vi "Initialize.vi"(8 "error in (no error)":errorcluster, 9 "GRR Data Mgr":string, 10 "Test Data Mgr":string, 11 "Result Display in":refnum<class "Result Display.lvclass">) -> (0 "error out":errorcluster, 3 "Result Display out":refnum<class "Result Display.lvclass">)   [LabVIEW 2018, in "Result Display.lvclass"]
uses:
  Result Display.lvclass
  Result Display.lvclass/Result Display.ctl
  TestDataMgr/TestDataMgr.lvclass
  Result Data Mgr/Result Data Mgr.lvclass
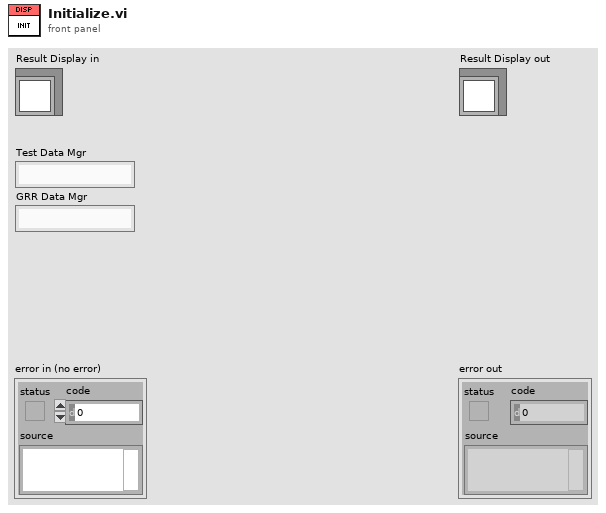
[diagram p1: front panel]
types:
  T1 = typedef "TestDataMgr.lvclass/Session Handle.ctl" = refnum<data-value>
  T2 = typedef "Result Data Mgr.lvclass/Session Handle.ctl" = refnum<data-value>
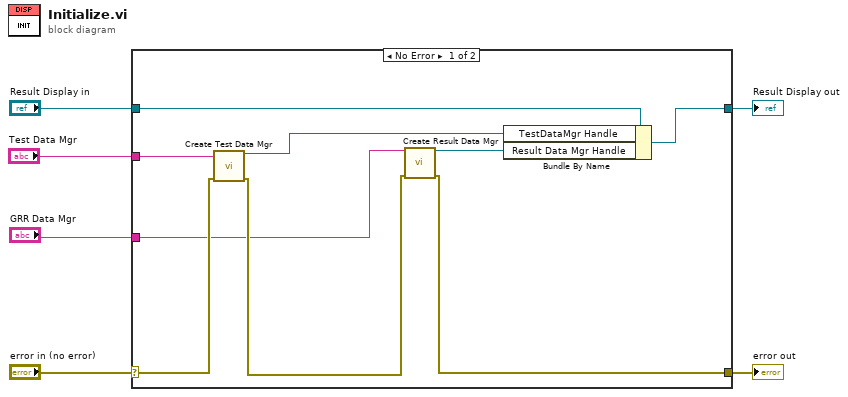
[diagram p0: block diagram]
diagram:
  n1 = case shown="No Error" "error in (no error)" {
    selector: "error in (no error)" -> [w12 w17]
    tunnel: [w10 w17] -> w5
    tunnel: [w7 w16] -> w3
    tunnel: "Result Display in" -> [w13 w16]
    tunnel: "Test Data Mgr" -> [w9 _]
    tunnel: "GRR Data Mgr" -> [w8 _]
    frame No Error {
      n2 = call "Create Test Data Mgr.vi"("Session  Name ()"=w9, "error in (no error)"=w12) -> ("Session Handle"=w15:T1, "error out"=w11:errorcluster)  [unwired: 12 in]
      n3 = call "Create Result Data Mgr.vi"("Session  Name ()"=w8, "error in (no error)"=w11) -> ("Session Handle"=w14:T2, "error out"=w10:errorcluster)  [unwired: 12 in]
      n4 = Bundle By Name(cluster=w13, "TestDataMgr Handle"=w15, "Result Data Mgr Handle"=w14) -> (w7:refnum<class "Result Display.lvclass">)
    }
    frame Error {
    }
  }
  "error out" <- w5
  "Result Display out" <- w3
